vi "SMC_RefMove.vi"(8 "error in (no error)":errorcluster, 11 "Number of revolutions":u8=10) -> (0 "error out":errorcluster)   [LabVIEW 2015]
uses:
  SMC_SubVIs.llb/SMC_ManagerMode.ctl
  SMC_SubVIs.llb/glb_stop.vi
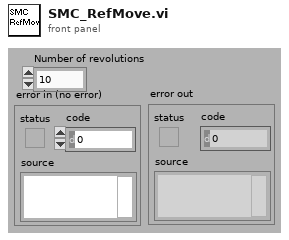
[diagram p1: front panel]
types:
  T1 = typedef "SMC_ManagerMode.ctl" = enum16{"Init", "Get", "SetPosition", "SetStatus", "SetMoving", "SetControllerNr"}
  T2 = typedef "SMC Paras.ctl" = cluster{"VENUS Language":T3, "Number of Axis":u8, "Controller Nr":u8, "Simulation":bool}
  T3 = typedef "VENUSNr.ctl" = enum16{"VENUS 2", "VENUS 1"}
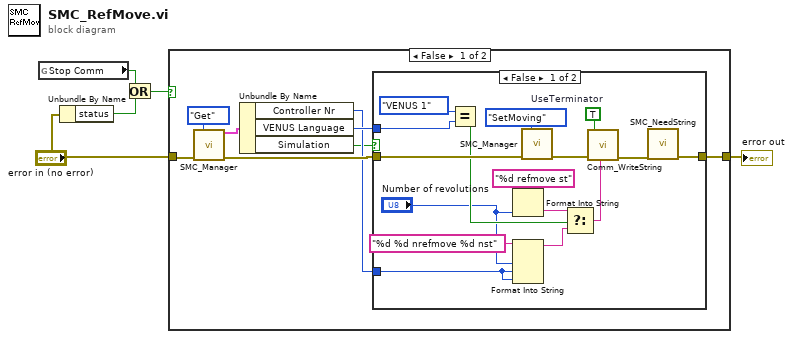
[diagram p0: block diagram]
diagram:
  n1 = global read "glb_stop.vi" "Stop Comm"() -> (w3:bool)
  n2 = Unbundle By Name("error in (no error)") -> ("status"=w1:bool)
  n3 = Or(x=w3, y=w1) -> (x .or. y?=w2:bool)
  n4 = case shown="False" w2 {
    tunnel: "error in (no error)" -> [w10 w31]
    tunnel: [w12 w31] -> w4
    frame False {
      n5 = call "SMC_Manager.vi"("Mode"=SMC_ManagerMode."Get", "error in (no error)"=w10) -> ("SMC Parameter Out"=w9:T2, "error out"=w11:errorcluster)  [unwired: 9 in, 3 out]
      n6 = Unbundle By Name(w9) -> ("Controller Nr"=w7:u8, "VENUS Language"=w8:T3, "Simulation"=w6:bool)
      n7 = case shown="False" w6 {
        tunnel: [w27 w30] -> w12
        tunnel: w11 -> [w26 w30]
        tunnel: w8 -> [w23 _]
        tunnel: w7 -> [w15 _]
        frame False {
          w14 = TRUE  # UseTerminator
          n8 = Equal?(x=enum16{"VENUS 2", "VENUS 1"}."VENUS 1", y=w23) -> (x = y?=w22:bool)
          n9 = Format Into String(format string="%d refmove st" ("Format String"), "Number of revolutions") -> (resulting string=w20:string)  [unwired: 2 in, 1 out]
          n10 = Format Into String(format string="%d %d nrefmove %d nst" ("Format String"), "Number of revolutions", w15, w15) -> (resulting string=w17:string)  [unwired: 2 in, 1 out]
          n11 = call "SMC_Manager.vi"("Mode"=SMC_ManagerMode."SetMoving", "error in (no error)"=w26) -> ("error out"=w25:errorcluster)  [unwired: 9 in, 4 out]
          n12 = Select(t=w20, s=w22, f=w17) -> (s? t:f=w18:string)
          n13 = call "Comm_WriteString.vi"("string to write"=w18, "error in (no error)"=w25, "UseTerminator"=w14) -> ("error out"=w28:errorcluster)  [unwired: 8 in]
          n14 = call "SMC_NeedString.vi"("error in (no error)"=w28) -> ("error out"=w27:errorcluster)  [unwired: 9 in, 1 out]
        }
        frame True {
          # "Simulation"
        }
      }
    }
    frame True {
      # "Error, do nothing"
    }
  }
  "error out" <- w4
